vi "LarAlignmentSource.vi"(2 "Level":i32=20, 9 "error in (no error)":errorcluster) -> (6 "error out":errorcluster)   [LabVIEW 2009]
uses:
  <vilib>/Instr/_visa.llb/VISA Configure Serial Port (Instr).vi
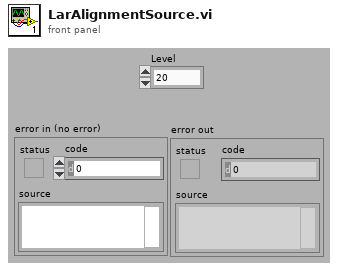
[diagram p1: front panel]
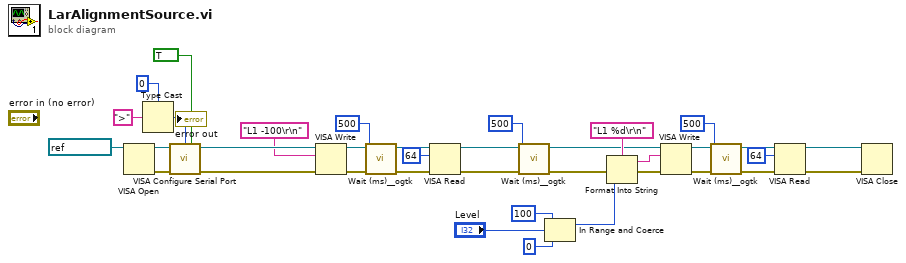
[diagram p0: block diagram]
diagram:
  n1 = VISA Open(VISA resource name=refnum<visa-resource-name> "COM53") -> (VISA resource name=w32:refnum<visa-resource-name>, error out=w31:errorcluster)  [unwired: 4 in]
  n2 = Type Cast(type=u8 0, x=">") -> (*(type *) &x=w28:u8)
  n3 = call-poly "VISA Configure Serial Port"("VISA resource name"=w32, "termination char\n(0xA = '\\n' = LF)"=w28, "Enable Termination\nChar (T)"=TRUE ("Enable Termination\nChar (T)"), "error in (no error)"=w31) -> ("VISA resource name out"=w7:refnum<visa-resource-name>, "error out"=w5:errorcluster)  [unwired: 10 in]
  n4 = VISA Write(VISA resource name=w7, write buffer="L1 -100\r\n" ("chaîne de format"), error in (no error)=w5) -> (VISA resource name out=w11:refnum<visa-resource-name>, error out=w8:errorcluster)  [unwired: 1 out]
  n5 = call <userlib>:"Wait (ms)__ogtk.vi"("error in (no error)"=w8, "milliseconds to wait"=u32 500) -> ("error out"=w10:errorcluster)  [unwired: 8 in, 1 out]
  n6 = VISA Read(VISA resource name=w11, byte count=u32 64, error in (no error)=w10) -> (VISA resource name out=w6:refnum<visa-resource-name>, error out=w2:errorcluster)  [unwired: 2 out]
  n7 = call <userlib>:"Wait (ms)__ogtk.vi"("error in (no error)"=w2, "milliseconds to wait"=u32 500) -> ("error out"=w1:errorcluster)  [unwired: 8 in, 1 out]
  n8 = In Range and Coerce(upper limit=100, x="Level", lower limit=0) -> (coerced(x)=w20:i32)  [unwired: 1 out]
  n9 = Format Into String(format string="L1 %d\r\n" ("chaîne de format"), error in=w1, w20) -> (resulting string=w24:string, error out=w25:errorcluster)  [unwired: 1 in]
  n10 = VISA Write(VISA resource name=w6, write buffer=w24, error in (no error)=w25) -> (VISA resource name out=w16:refnum<visa-resource-name>, error out=w19:errorcluster)  [unwired: 1 out]
  n11 = call <userlib>:"Wait (ms)__ogtk.vi"("error in (no error)"=w19, "milliseconds to wait"=u32 500) -> ("error out"=w17:errorcluster)  [unwired: 8 in, 1 out]
  n12 = VISA Read(VISA resource name=w16, byte count=u32 64, error in (no error)=w17) -> (VISA resource name out=w14:refnum<visa-resource-name>, error out=w13:errorcluster)  [unwired: 2 out]
  n13 = VISA Close(VISA resource name=w14, error in (no error)=w13) -> ()  [unwired: 1 out]
